vi "Set Cell Value.vi"(6 "Value":variant, 8 "error in":errorcluster, 9 "Column":i32, 10 "Row":i32, 11 "SourceGrid in":refnum<class "SourceGrid.lvclass">) -> (0 "error out":errorcluster, 3 "SourceGrid out":refnum<class "SourceGrid.lvclass">)   [LabVIEW 2023, in "SourceGrid.lvlib" / "SourceGrid.lvclass"]
uses:
  SourceGrid.lvclass
  SourceGrid.lvclass/SourceGrid.ctl
  Cells/Cell/Cell.lvclass
  Cells/Check Box/Check Box.lvclass
  D:/git/Sourcegrid-LabVIEW/source/Cells/Cell/Cell.lvclass
  Cells/Image/Image.lvclass
  D:/git/Sourcegrid-LabVIEW/dll/SourceGrid.dll
  dll/SourceGrid.dll
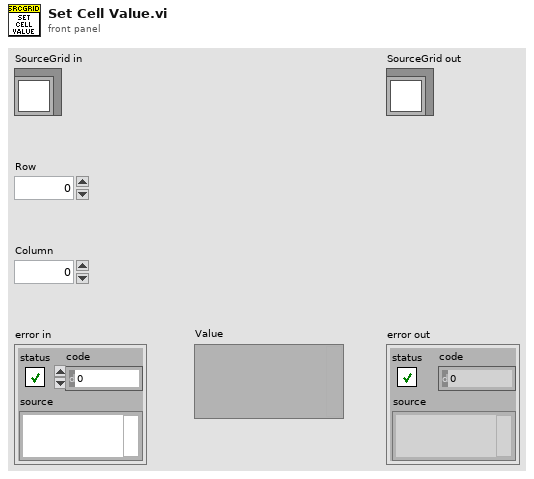
[diagram p1: front panel]
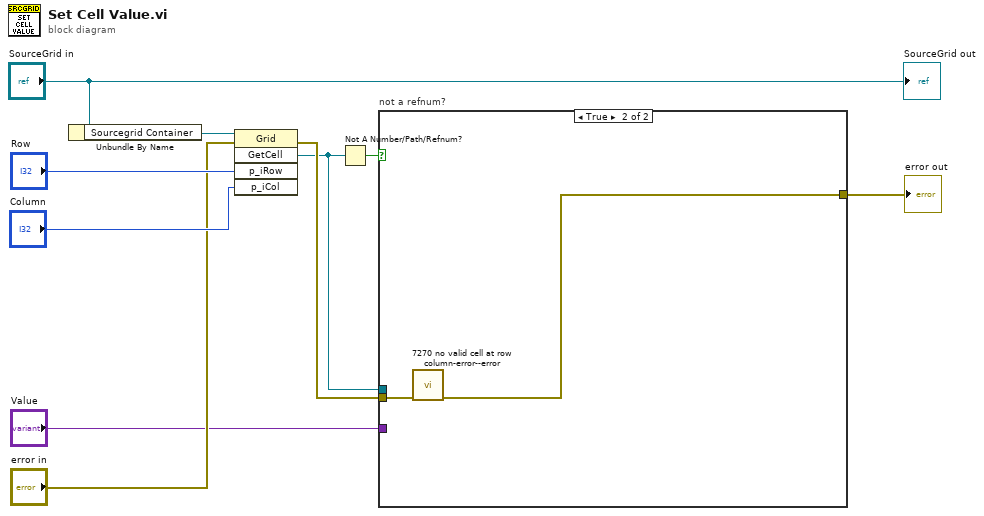
[diagram p0: block diagram]
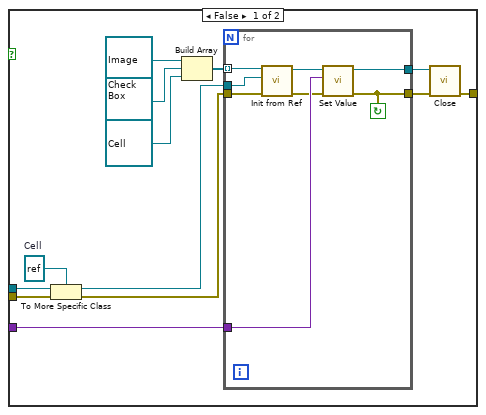
[diagram p2: hidden frame]
diagram:
  n1 = Unbundle By Name("SourceGrid in") -> ("Sourcegrid Container"=w9:refnum<k24>)
  n2 = invoke class="Grid" method="GetCell"(reference=w9, error in="error in", "p_iRow"="Row", "p_iCol"="Column") -> (error out=w6:errorcluster, "GetCell"=w1:refnum<k24>)  [unwired: 1 in, 3 out]
  n3 = Not A Number/Path/Refnum?(number/path/refnum=w1) -> (NaN/Path/Refnum?=w2:bool)
  n4 = case "not a refnum?" shown="True" w2 {
    tunnel: w1 -> [w22 _]
    tunnel: w6 -> [w21 w33]
    tunnel: "Value" -> [w14 _]
    tunnel: [w11 w32] -> w3
    frame False {
      w23 = refnum<k24> refnum  # Cell
      n5 = To More Specific Class(target class=w23, reference=w22, error in=w21) -> (specific class reference=w15:refnum<k24>, error out=w16:errorcluster)
      n6 = Build Array(refnum<class "Image.lvclass"> refnum ("SourceGrid.lvlib:Check Box"), refnum<class "Check Box.lvclass"> refnum ("SourceGrid.lvlib:Check Box"), refnum<class "Cell.lvclass"> refnum ("SourceGrid.lvlib:Cell")) -> (w17:refnum<class "Cell.lvclass">[])
      n7 = for {
        tunnel: w17 -> [w31] mode=indexing
        tunnel: w15 -> [w24]
        tunnel: w14 -> [w28]
        tunnel: [w26] -> w12
        tunnel: w16 -> [w30]
        tunnel: [w25] -> w13
        stop <- w25 continue-if-true
        n8 = call-dynamic "Init from Ref.vi"("error in"=w30, "Cell"=w24, "Cell in"=w31) -> ("error out"=w27:errorcluster, "Cell out"=w29:refnum<class "Cell.lvclass">)  [unwired: 7 in]
        n9 = call-dynamic "Set Value.vi"("error in"=w27, "Value"=w28, "Cell in"=w29) -> ("error out"=w25:errorcluster, "Cell out"=w26:refnum<class "Cell.lvclass">)  [unwired: 7 in]
      }
      n10 = call-dynamic "Close.vi"("error in"=w13, "Cell in"=w12) -> ("error out"=w11:errorcluster)  [unwired: 8 in, 1 out]
    }
    frame True {
      n11 = call "7270 no valid cell at row column-error--error.vi"("error in"=w33) -> ("error out"=w32:errorcluster)  [unwired: 10 in]
    }
  }
  "error out" <- w3
  "SourceGrid out" <- "SourceGrid in"
